vi "Get Magnet Field.vi"(0 "Z-Axis Communications Config":T1={"GPIB address"=22, "GPIB bus"=0, "connection ID"=refnum, "IP"="111.111.111.1", "Active Comm Interface"=0, "Serial Port"="", "Programmer Type"=0} {"Programmer Type" items=["Model 430", "Model 420"]; "Active Comm Interface" items=["TCP/IP (Model 430 Only)", "RS232", "IEEE488"]}, 1 "error in":T2) -> (2 "Magnet Field (kG)":dbl format="%.3f", 3 "Instrument Responded?":bool, 4 "error out":T2)   [LabVIEW 2018]
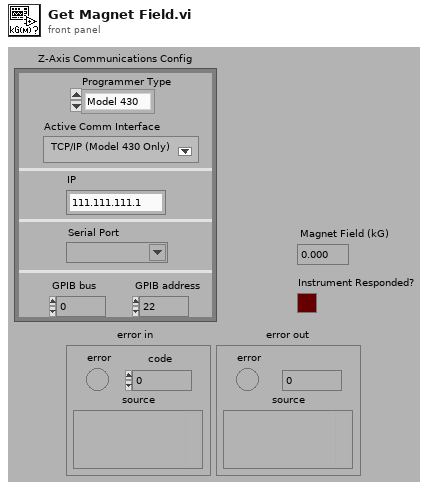
[diagram p1: front panel]
types:
  T1 = cluster{"GPIB address":i16, "GPIB bus":i16, "connection ID":refnum<k5>, "IP":string, "Active Comm Interface":u16, "Serial Port":refnum<visa-resource-name>, "Programmer Type":u16}
  T2 = cluster{"error":bool, "code":i32, "source":string}
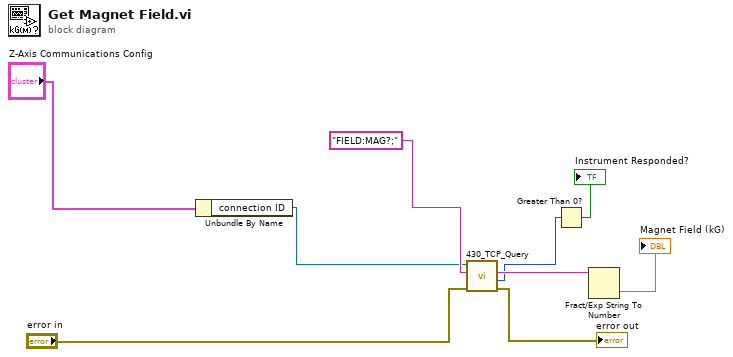
[diagram p0: block diagram]
diagram:
  n1 = Unbundle By Name("Z-Axis Communications Config") -> ("connection ID"=w1:refnum<k5>)
  n2 = call "430_TCP_Query.vi"("error in (no error)"="error in", "Command"="FIELD:MAG?;", "connection ID"=w1) -> ("error out"=→"error out":errorcluster, "Bytes Read"=w3:i32, "Response"=w4:string)  [unwired: 4 in, 2 out]
  n3 = Greater Than 0?(x=w3) -> (x > 0?=→"Instrument Responded?":bool)
  n4 = Fract/Exp String To Number(string=w4) -> (number=→"Magnet Field (kG)":dbl)  [unwired: 3 in, 1 out]
